vi "Insert Element at Start.vi"(8 "error in (no error)":errorcluster, 9 "element":variant, 10 "Name":string, 11 "Variant (Cluster) in":variant) -> (0 "error out":errorcluster, 3 "Variant (Cluster) out":variant)   [LabVIEW 2017, in "Advanced Variant Tools.lvlib"]
uses:
  Advanced Variant Tools.lvlib
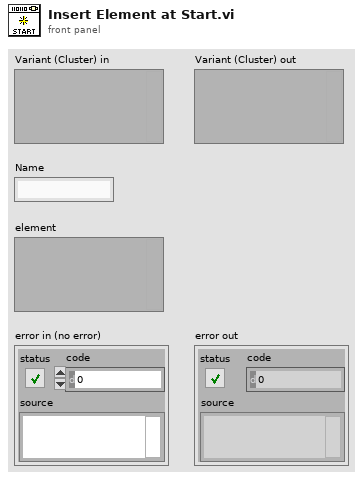
[diagram p1: front panel]
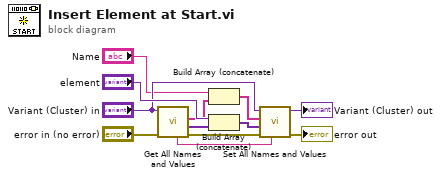
[diagram p0: block diagram]
diagram:
  n1 = call "Get All Names and Values.vi"("error in"="error in (no error)", "Cluster In"="Variant (Cluster) in") -> ("error out"=w10:errorcluster, "Values"=w11:variant[], "Item Names"=w4:string[], "Name"=w1:string)  [unwired: 5 in, 1 out]
  n2 = Build Array (concatenate)("Name", w4) -> (w2:string[])
  n3 = Build Array (concatenate)("element", w11) -> (w7:variant[])
  n4 = call "Set All Names and Values.vi"("Name"=w1, "error in"=w10, "values"=w7, "Item Names"=w2, "Cluster In"="Variant (Cluster) in") -> ("error out"=→"error out":errorcluster, "Cluster Out"=→"Variant (Cluster) out":variant)  [unwired: 5 in]
